vi "Vision Processing.vi"(4 "error in (no error)":errorcluster) -> ()   [LabVIEW 2014]
doc: "This VI runs in parallel to other tasks. It gets images from the camera, processes them for color or shape and use that information to affect robot behavior."
uses:
  <vilib>/Rock Robotics/SystemInterfaces/NetworkCommunication/NetComm_UsageReport_ResourceType.ctl
  <vilib>/Rock Robotics/Network Tables/SD Read Boolean.vi
  Robot Global Data.vi
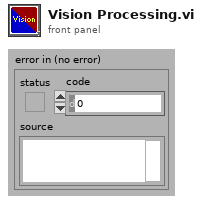
[diagram p1: front panel]
types:
  T1 = cluster{"fps":i32, "compression":i32, "compression 2":i32}
  T2 = typedef "NetComm_UsageReport_ResourceType.ctl" = enum8{"Controller", "Module", "Language", "CANPlugin", "Accelerometer", "ADXL345", "AnalogChannel", "AnalogTrigger", "AnalogTriggerOutput", "CANJaguar", "Compressor", "Counter", "Dashboard", "DigitalInput", "DigitalOutput", "DriverStationCIO", "DriverStationEIO", "DriverStationLCD", "Encoder", "GearTooth", "Gyro", "I2C", "Framework", "Jaguar", "Joystick", "Kinect", "KinectStick", "PIDController", "Preferences", "PWM", "Relay", "RobotDrive", "SerialPort", "Servo", "Solenoid", "SPI", "Task", "Ultrasonic", "Victor", "Button", "Command", "AxisCamera", "PCVideoServer", "SmartDashboard", "Talon", "HiTechnicColorSensor", "HiTechnicAccel", "HiTechnicCompass", "SRF08", "AnalogOutput", "Victor SP", "Talon SRX", "CAN Talon SRX"}
  T3 = enum16{"Update Mode", "Get Image", "Get Image Data"}
  T4 = typedef "WPI_CameraDevRef.ctl" = cluster{"Camera Address":string, "CameraStatus":errorcluster}
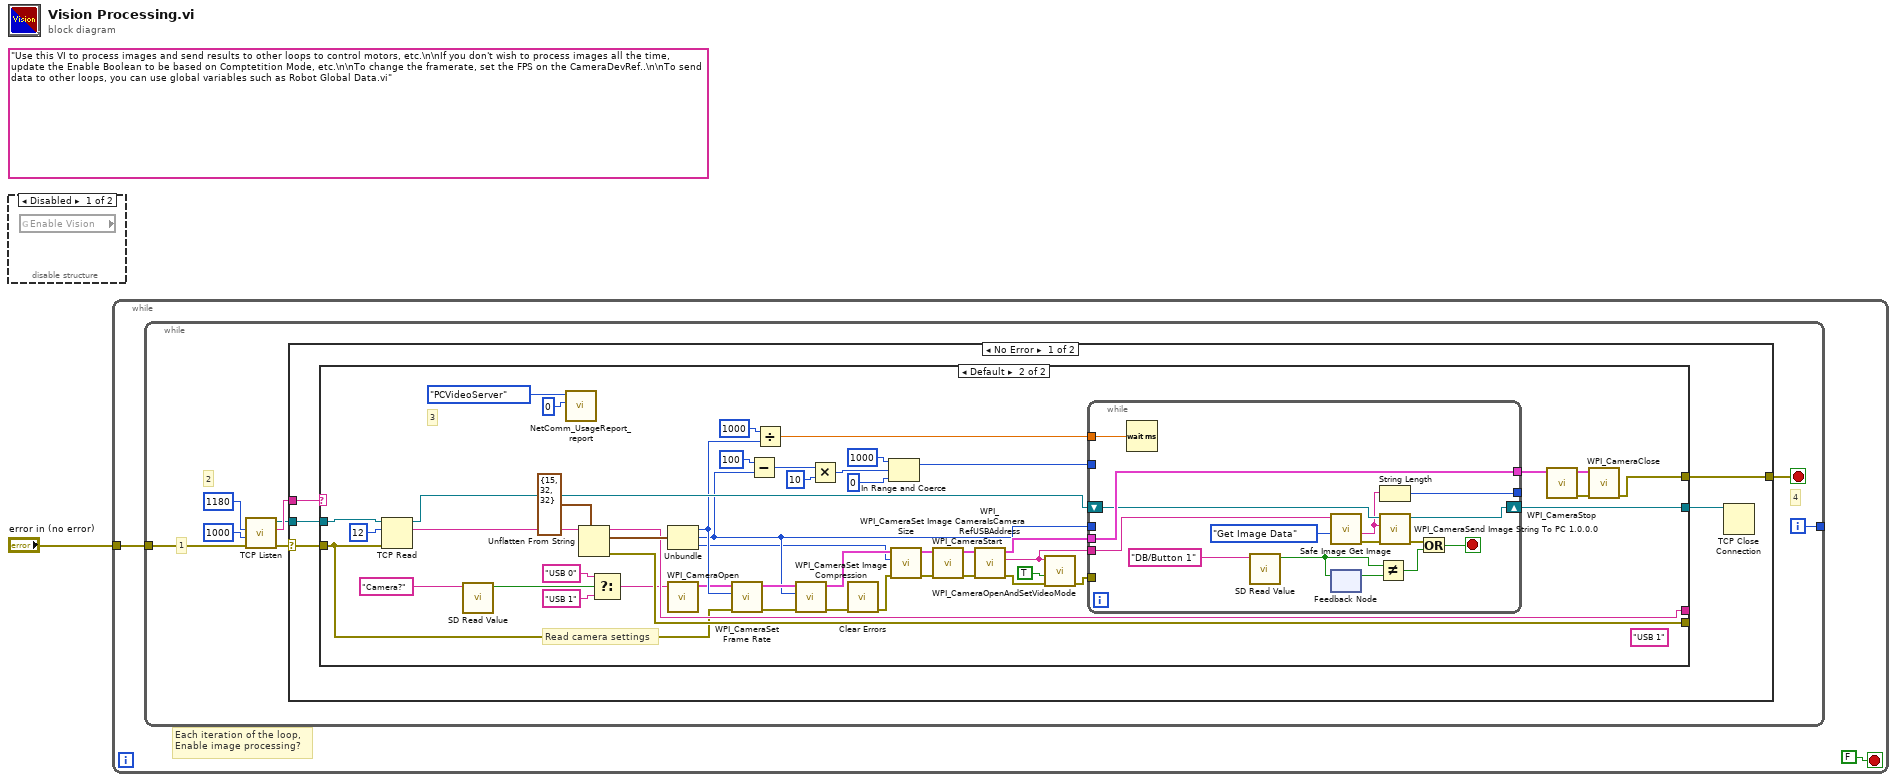
[diagram p0: block diagram]
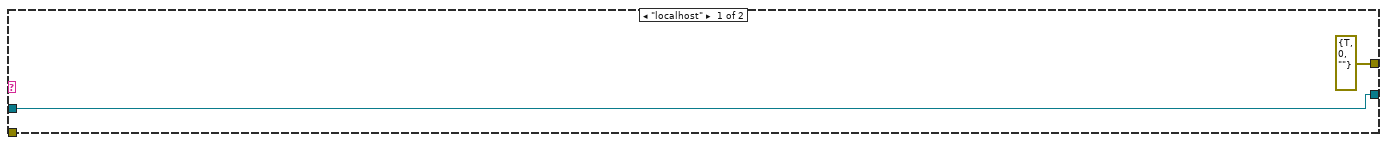
[diagram p3: hidden frame]
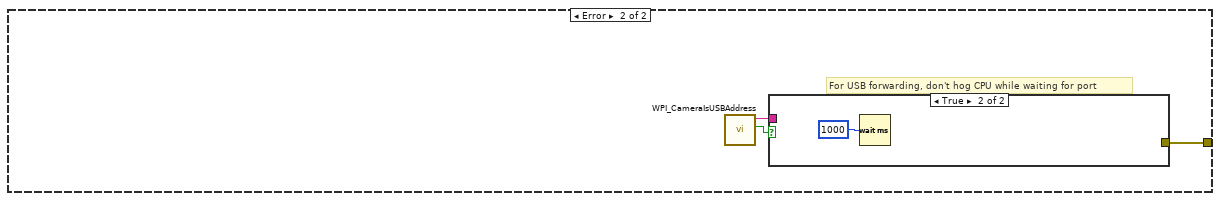
[diagram p4: hidden frame]
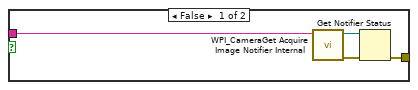
[diagram p5: hidden frame]
diagram:
  (unwired) "Use this VI to process images and send results to other loops to control motors, etc.\n\nIf you don't wish to process images all the time, update the Enable Boolean to be based on Comptetition Mode, etc.\n\nTo change the framerate, set the FPS on the CameraDevRef..\n\nTo send data to other loops, you can use global variables such as Robot Global Data.vi"
  n1 = disable-structure shown="Disabled" {
    frame Disabled {
      n2 = global read "Robot Global Data.vi" "Enable Vision"() -> ()  [unwired: 1 out]
    }
    frame Enabled {
    }
  }
  n3 = while {
    tunnel: "error in (no error)" -> [w2]
    stop <- FALSE stop-if-true
    # "Each iteration of the loop,\nEnable image processing?"
    n4 = while {
      tunnel: w2 -> [w10]
      tunnel: [w4] -> _
      i -> [w4]
      stop <- w8 stop-if-true
      # "4"
      # "1"
      # "2"
      n5 = call <vilib>:"TCP Listen.vi"("error in (no error)"=w10, "timeout ms (wait forever: -1)"=u16 1000 ("port"), "port"=u16 1180) -> ("error out"=w6:errorcluster, "remote address"=w11:string, "connection ID"=w9:refnum<k5>)  [unwired: 1 in, 5 out]
      n6 = case shown="No Error" w6 {
        selector: w6 -> [w12 _]
        tunnel: w11 -> [w16 _]
        tunnel: w9 -> [w15 _]
        tunnel: [w14 w84] -> w8
        frame No Error {
          n7 = case shown="Default" w16 {
            tunnel: w12 -> [_ w33]
            tunnel: w15 -> [w17 w57]
            tunnel: [errorcluster {"status"=TRUE, "code"=0, "source"=""} ("error out 2") w19] -> w14
            tunnel: [w17 w66] -> w13
            tunnel: [_ w35] -> _
            tunnel: [_ w34] -> _
            frame "localhost" {
            }
            frame Default {
              (unwired) "USB 1" ("format string")
              # "Read camera settings"
              # "3"
              n8 = TCP Read(connection ID=w57, bytes to read=12, error in (no error)=w33) -> (connection ID out=w56:refnum<k5>, data out=w54:string)  [unwired: 2 in, 1 out]
              n9 = call-poly <vilib>:"SD Read Value.vi"("Name"="Camera?") -> ("Boolean"=w26:bool)  [unwired: 8 in, 2 out]
              n10 = call <vilib>:"NetComm_UsageReport_report.vi"("Instance Number"=u8 0, "Resource Type"=NetComm_UsageReport_ResourceType."PCVideoServer") -> ()  [unwired: 10 in]
              n11 = Unflatten From String(type=T1 {"fps"=15, "compression"=32, "compression 2"=32} ("Camera Settings"), binary string=w54) -> (rest of the binary string=w34:string, value=w48:T1, error out=w35:errorcluster)  [unwired: 3 in]
              n12 = Select(t="USB 0" ("format string"), s=w26, f="USB 1" ("format string")) -> (s? t:f=w21:string)
              n13 = Unbundle(w48) -> ("fps"=w32:i32, "compression"=w31:i32, "compression 2"=w30:i32)
              n14 = call <vilib>:"WPI_CameraOpen.vi"("Camera Address"=w21) -> ("CameraDevRef"=w20:T4)  [unwired: 1 in, 9 out]
              n15 = call <vilib>:"WPI_CameraSet Frame Rate.vi"("error in (no error)"=w33, "Frame Rate (fps)"=w32, "CameraDevRef"=w20) -> ("error out"=w50:errorcluster, "CameraDevRef Out"=w53:T4)  [unwired: 7 in]
              n16 = Subtract(x=100, y=w31) -> (x-y=w41:i32)
              n17 = Divide(x=u16 1000 ("port"), y=w32) -> (x/y=w46:dbl)
              n18 = call <vilib>:"WPI_CameraSet Image Compression.vi"("error in (no error)"=w50, "Compression"=w31, "CameraDevRef"=w53) -> ("error out"=w37:errorcluster, "CameraDevRef Out"=w52:T4)  [unwired: 7 in]
              n19 = Multiply(x=w41, y=10) -> (x*y=w43:i32)
              n20 = call <vilib>:"Clear Errors.vi"("error in (no error)"=w37) -> ("error out"=w36:errorcluster)  [unwired: 5 in, 1 out]
              n21 = In Range and Coerce(upper limit=1000, x=w43, lower limit=0) -> (coerced(x)=w39:i32)  [unwired: 1 out]
              n22 = call <vilib>:"WPI_CameraSet Image Size.vi"("error in (no error)"=w36, "Image Size"=w30, "CameraDevRef"=w52) -> ("error out"=w49:errorcluster, "CameraDevRef Out"=w51:T4)  [unwired: 7 in]
              n23 = call <vilib>:"WPI_CameraStart.vi"("error in (no error)"=w49, "CameraDevRef"=w51) -> ("error out"=w61:errorcluster, "CameraDevRef Out"=w59:T4)  [unwired: 8 out]
              n24 = call <vilib>:"WPI_CameraIsCameraRefUSBAddress.vi"("error in (no error)"=w61, "CameraDevRef"=w59) -> ("error out"=w60:errorcluster, "Camera Address Out"=w62:string, "CameraDevRef out"=w58:T4)  [unwired: 6 in, 1 out]
              n25 = call <vilib>:"WPI_CameraOpenAndSetVideoMode.vi"("error in (no error)"=w60, "USB JPEG"=TRUE, "Camera Address Out"=w62) -> ("error out"=w29:errorcluster)  [unwired: 8 in]
              n26 = while {
                tunnel: w62 -> [w67]
                shift-right: [w81] -> w66
                shift-left: w56 -> [w78]
                tunnel: [w80] -> w65
                tunnel: w58 -> [w80]
                tunnel: w39 -> [_]
                tunnel: w46 -> [w79]
                tunnel: [w77] -> _
                tunnel: w31 -> [_]
                tunnel: w29 -> [_]
                stop <- w68 stop-if-true
                n27 = Wait (ms)(milliseconds to wait=w79) -> ()  [unwired: 1 out]
                n28 = call-poly <vilib>:"SD Read Value.vi"("Name"="DB/Button 1") -> ("Boolean"=w71:bool)  [unwired: 8 in, 2 out]
                n29 = call <vilib>:"Safe Image Get Image.vi"("Operation"=T3."Get Image Data", "Session In"=w67) -> ("error out"=w73:errorcluster, "Image Data String"=w74:string)  [unwired: 6 in, 2 out]
                n30 = feedback-in #1(w71) -> ()
                n31 = feedback #1() -> (w72:bool)  [unwired: 1 in]
                n32 = Not Equal?(x=w71, y=w72) -> (x != y?=w70:bool)
                n33 = String Length(string=w74) -> (length=w77:i32)
                n34 = call <vilib>:"WPI_CameraSend Image String To PC 1.0.0.0.vi"("error in (no error)"=w73, "String"=w74, "TCP Connection ID"=w78) -> ("error out"=w69:errorcluster, "TCP Connection ID out"=w81:refnum<k5>)  [unwired: 7 out]
                n35 = Or(x=w69, y=w70) -> (x .or. y?=w68:bool)
              }
              n36 = call <vilib>:"WPI_CameraStop.vi"("CameraDevRef"=w65) -> ("error out"=w24:errorcluster, "CameraDevRef Out"=w25:T4)  [unwired: 1 in, 8 out]
              n37 = call <vilib>:"WPI_CameraClose.vi"("error in (no error)"=w24, "CameraDevRef"=w25) -> ("error out"=w19:errorcluster)  [unwired: 9 in]
            }
          }
          n38 = TCP Close Connection(connection ID=w13) -> ()  [unwired: 1 in, 3 out]
        }
        frame Error {
          # "For USB forwarding, don't hog CPU while waiting for port"
          n39 = call <vilib>:"WPI_CameraIsUSBAddress.vi"() -> ("USB?"=w82:bool, "Camera Address Out"=w83:string)  [unwired: 9 in, 1 out]
          n40 = case shown="True" w82 {
            tunnel: [w88 _] -> w84
            tunnel: w83 -> [w85 _]
            frame False {
              n41 = call <vilib>:"WPI_CameraGet Acquire Image Notifier Internal.vi"("Camera Address"=w85) -> ("error out"=w86:errorcluster, "Acquire Image Notifier"=w87:refnum<notifier>)  [unwired: 1 in, 8 out]
              n42 = Get Notifier Status(notifier=w87, error in (no error)=w86) -> (error out=w88:errorcluster)  [unwired: 4 out]
            }
            frame True {
              n43 = Wait (ms)(milliseconds to wait=u32 1000) -> ()  [unwired: 1 out]
            }
          }
        }
      }
    }
  }
